vi "Get XML Inner Text.vi"(8 "error in":errorcluster, 9 "Tag":string, 11 "XML string":string) -> (0 "error out":errorcluster, 2 "Remaining Text":string, 3 "Inner Text":string, 4 "Not Found":bool)   [LabVIEW 2012]
uses:
  <vilib>/Utility/error.llb/whitespace.ctl
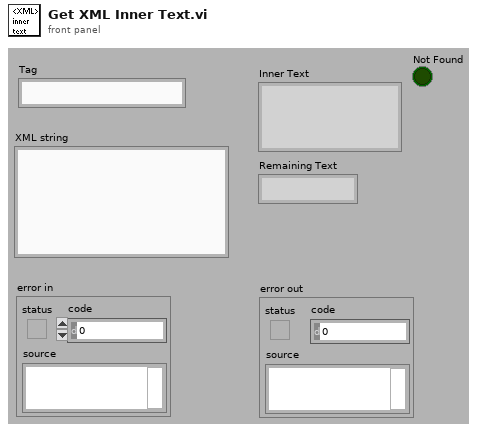
[diagram p1: front panel]
types:
  T1 = typedef "whitespace.ctl" = u16
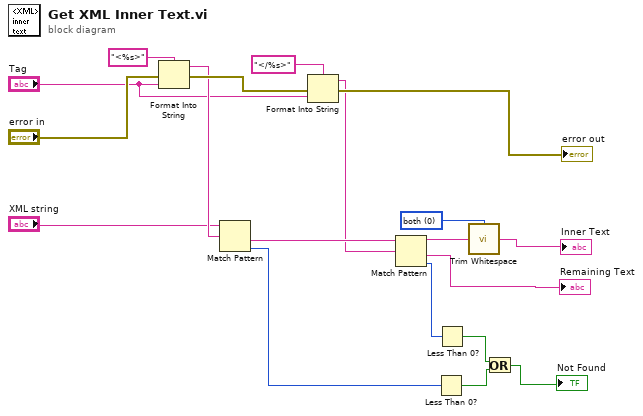
[diagram p0: block diagram]
diagram:
  w8 = T1 0 items=["both", "start of string", "end of string"] ("location (both)")
  n1 = Format Into String(format string="<%s>", error in="error in", "Tag") -> (resulting string=w15:string, error out=w17:errorcluster)  [unwired: 1 in]
  n2 = Match Pattern(string="XML string", regular expression=w15) -> (after substring=w16:string, offset past match=w9:i32)  [unwired: 1 in, 2 out]
  n3 = Format Into String(format string="</%s>", error in=w17, "Tag") -> (resulting string=w13:string, error out=→"error out":errorcluster)  [unwired: 1 in]
  n4 = Match Pattern(string=w16, regular expression=w13) -> (before substring=w7:string, after substring=→"Remaining Text":string, offset past match=w5:i32)  [unwired: 1 in, 1 out]
  n5 = Less Than 0?(x=w9) -> (x < 0?=w3:bool)
  n6 = Less Than 0?(x=w5) -> (x < 0?=w4:bool)
  n7 = call <vilib>:"Trim Whitespace.vi"("string"=w7, "location (both)"=w8) -> ("trimmed string"=→"Inner Text":string)
  n8 = Or(x=w4, y=w3) -> (x .or. y?=→"Not Found":bool)
